vi "test29-MappingRelationshipByExternalRegistration_State.vi"(8 "error in (no error)":errorcluster, 11 "TestCase in":refnum<class "testcase-CSMBroadcast.lvclass">) -> (0 "error out":errorcluster, 3 "TestCase out":refnum<class "testcase-CSMBroadcast.lvclass">)   [LabVIEW 2017, in "testcase-CSMBroadcast.lvclass"]
uses:
  testcase-CSMBroadcast.lvclass
  5f1321ef-d679-4204-8b32-271554a776bf.vi
  3afc563d-56e9-48a4-901d-19be23a22e68.vi
  src/user.lib/_NEVSTOP/Communicable State Machine(CSM)/AdvanceAPI/CSM - Revert Arguments-Safe String.vi
  src/user.lib/_NEVSTOP/Communicable State Machine(CSM)/AdvanceAPI/CSM - Make String Arguments Safe.vi
  src/user.lib/_NEVSTOP/Communicable State Machine(CSM)/AdvanceAPI/CSM - Break Down Multiple States String.vi
  src/user.lib/_NEVSTOP/Communicable State Machine(CSM)/AdvanceAPI/CSM - Keywords.vi
  src/user.lib/_NEVSTOP/Communicable State Machine(CSM)/_Polymophic/CSM - Replace Marks in Messages.vi
  src/user.lib/_NEVSTOP/Communicable State Machine(CSM)/_Shared/Trim Single-line Text.vi
  src/user.lib/_NEVSTOP/Communicable State Machine(CSM)/Communicable State Machine.lvlib
  <vilib>/addons/_JKI Toolkits/VI Tester/TestCase.llb/TestCase.lvclass
  C:/Program Files (x86)/National Instruments/LabVIEW 2017/vi.lib/addons/_JKI Toolkits/VI Tester/TestCase.llb/TestCase.lvclass
panel:
  out "State History 2":string
  out "Loop Count":i32
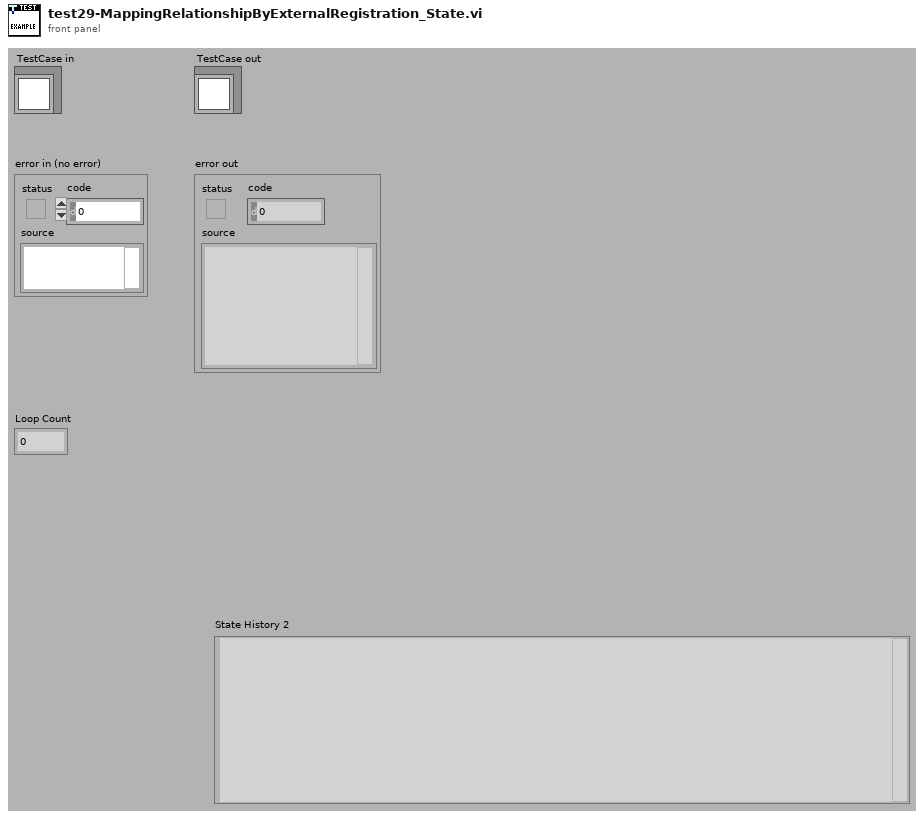
[diagram p1: front panel]
types:
  T1 = enum32{"Invalid", "Standard", "Closed", "Hidden", "Minimized", "Maximized"}
  T2 = enum32{"invalid app kind", "Development System", "Run Time System", "Student Edition", "Embedded LabVIEW", "Evaluation", "Custom"}
  T3 = cluster{"Status":string, "Source CSM":string, "Target CSM":string, "Target API":string}[]
  T4 = typedef "Communicable State Machine.lvlib/_CSM_Response Source Message.ctl" = cluster{"‘State":string, "’Arguments":string, "’Error":errorcluster}
  T5 = cluster{"Current VI Reference":refnum<vi>, "Close Panel on Exit?":bool}
  T6 = cluster{"Core":cluster{"Current VI Reference":refnum<vi>, "Close Panel on Exit?":bool}, "Your Boolean data":bool, "Your string data":string}
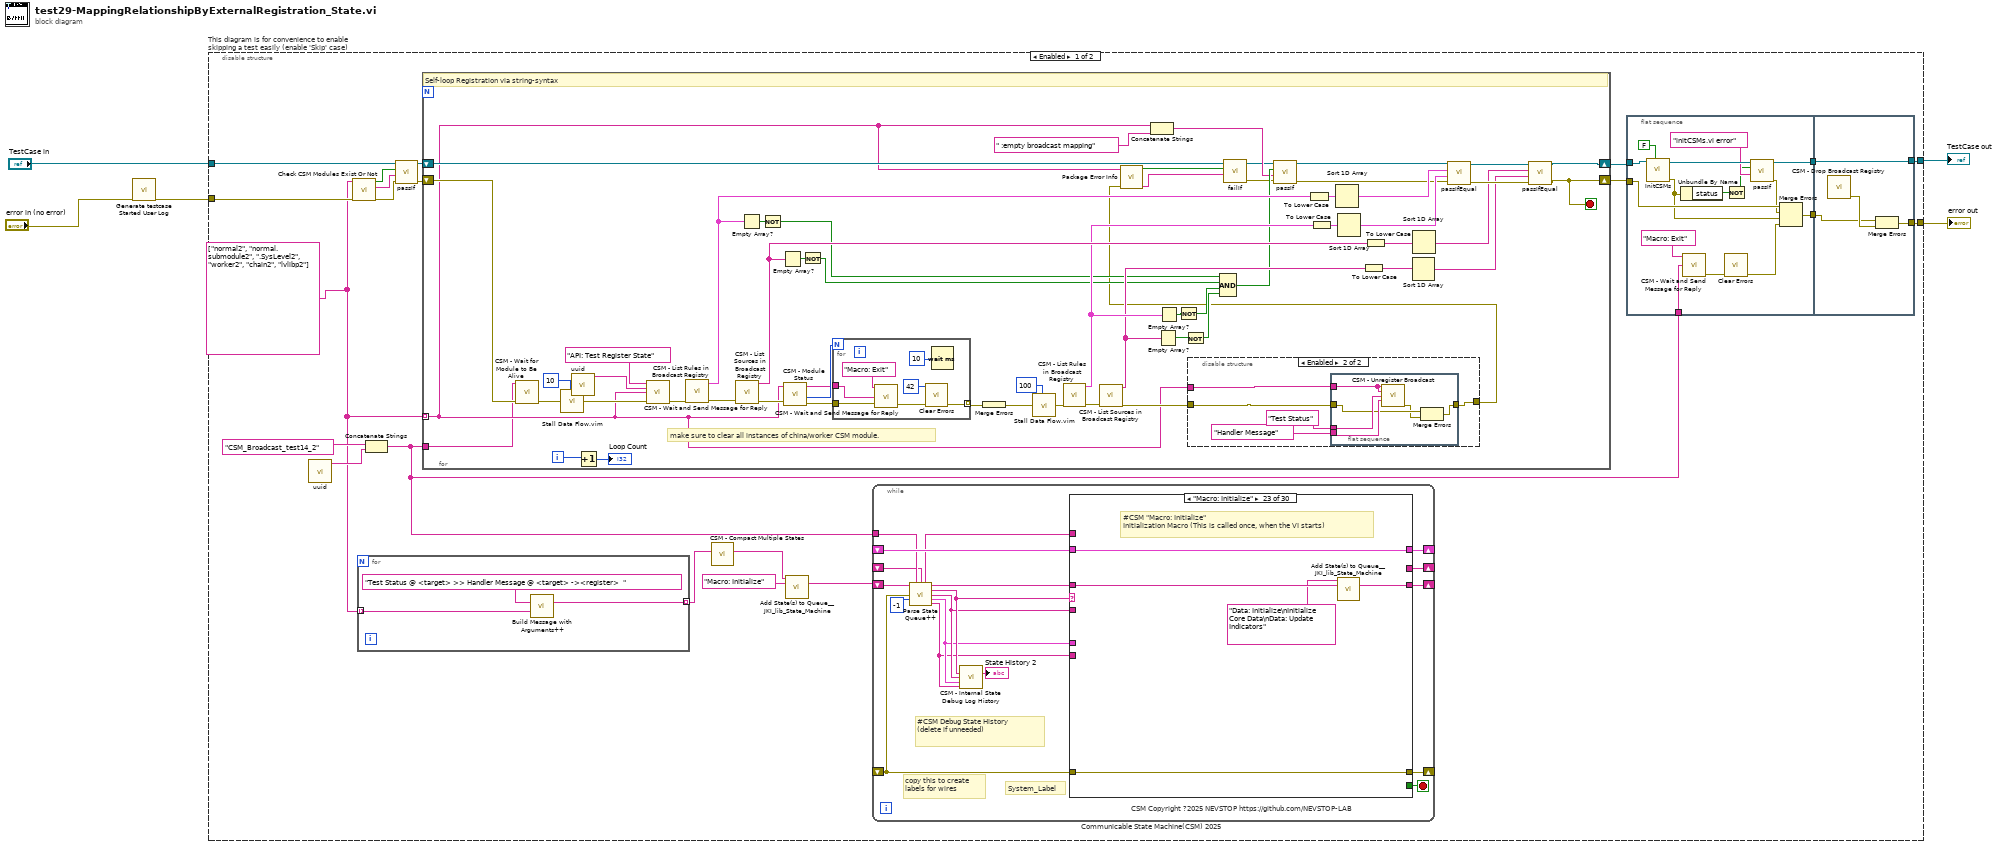
[diagram p0: block diagram]
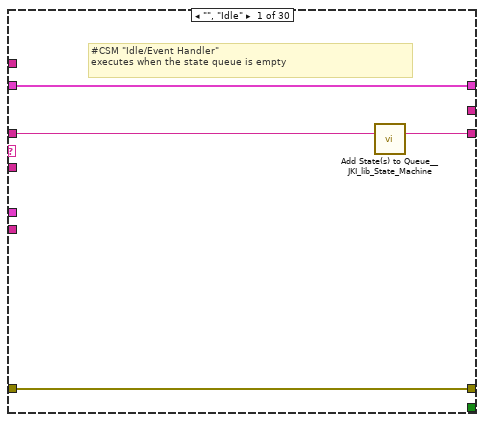
[diagram p2: hidden frame]
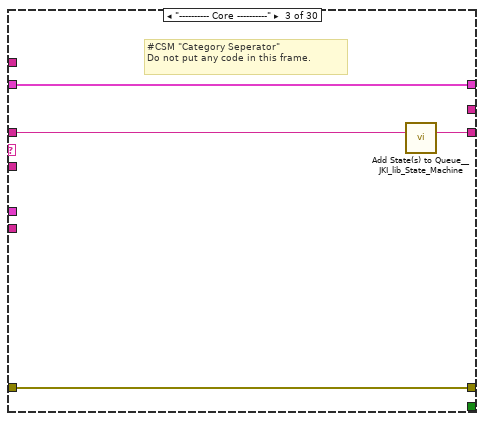
[diagram p4: hidden frame]
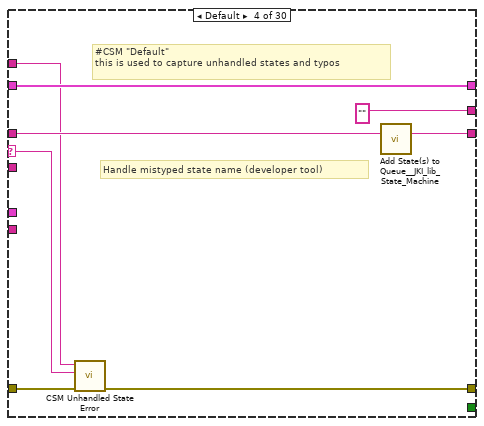
[diagram p5: hidden frame]
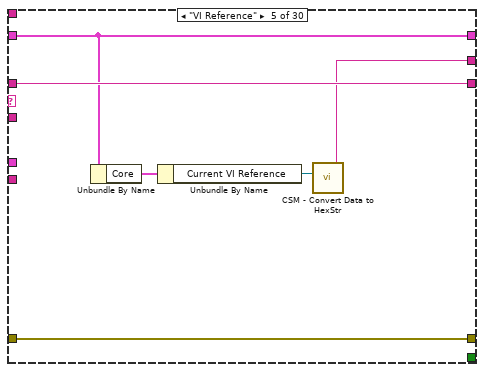
[diagram p6: hidden frame]
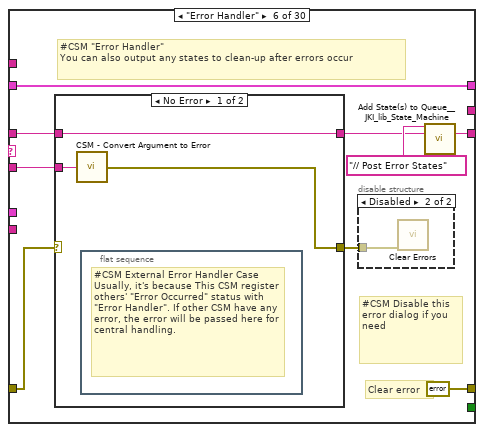
[diagram p7: hidden frame]
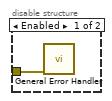
[diagram p8: hidden frame]
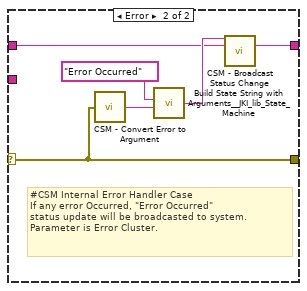
[diagram p9: hidden frame]
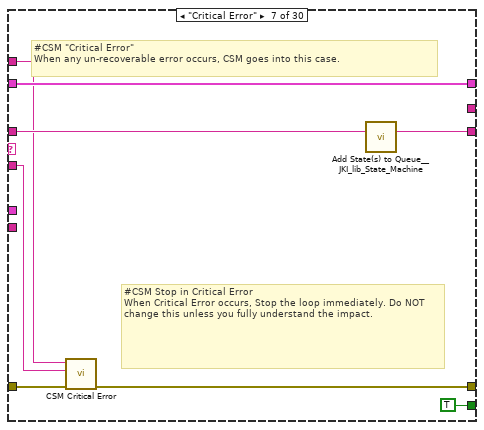
[diagram p10: hidden frame]
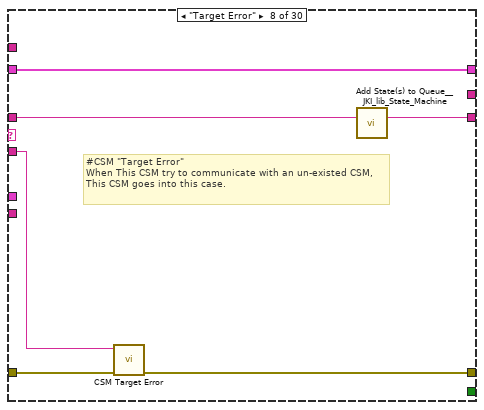
[diagram p11: hidden frame]
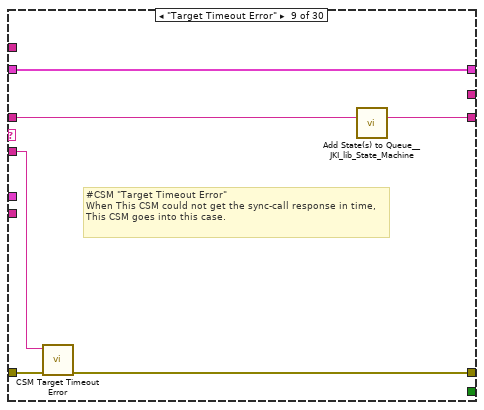
[diagram p12: hidden frame]
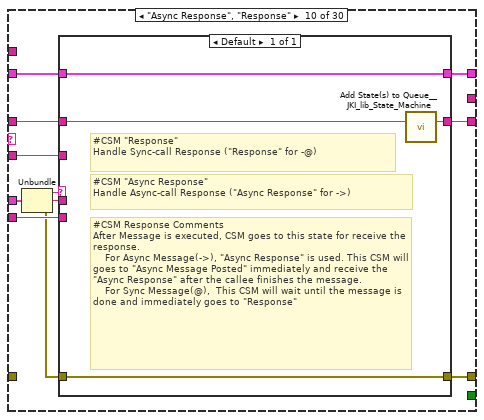
[diagram p13: hidden frame]
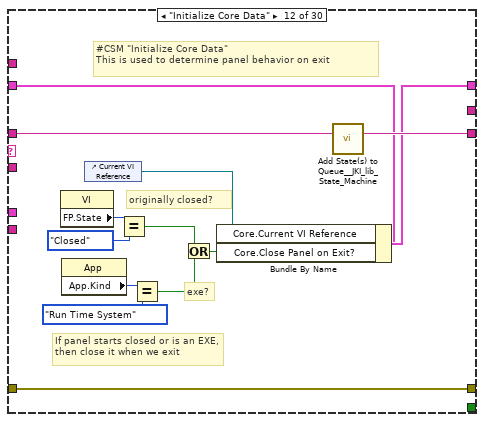
[diagram p15: hidden frame]
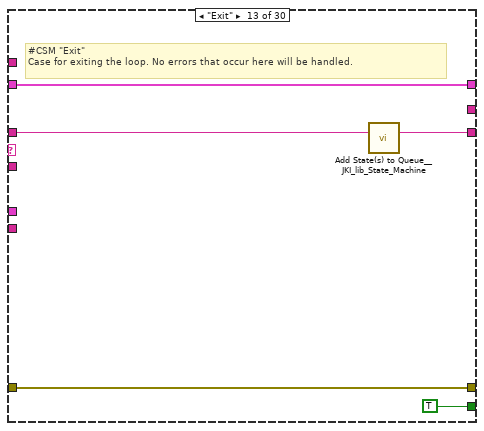
[diagram p16: hidden frame]
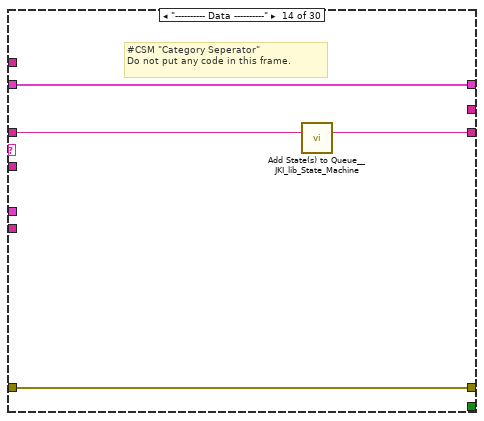
[diagram p17: hidden frame]
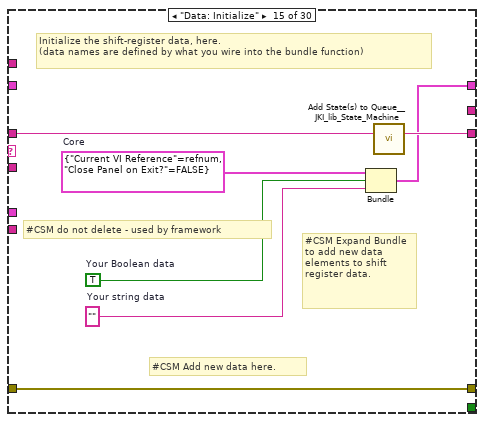
[diagram p18: hidden frame]
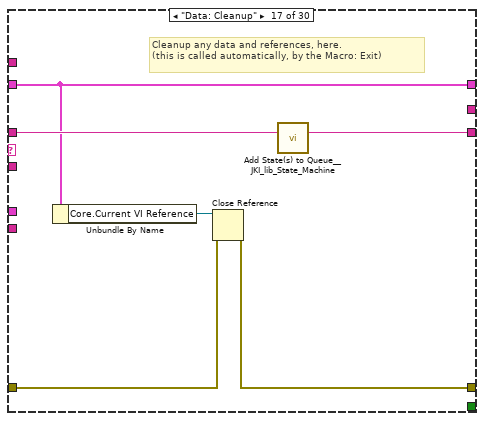
[diagram p20: hidden frame]
diagram:
  n1 = call "Generate testcase Started User Log.vi"("Error In"="error in (no error)") -> ("error out"=w1:errorcluster)  [unwired: 10 in]
  n2 = disable-structure "This diagram is for convenience to enable skipping a test easily (enable 'Skip' case)" shown="Enabled" {
    disable-tunnel: "TestCase in" -> [w21 w405]
    disable-tunnel: [w15 w403] -> w2
    disable-tunnel: [w14 w404] -> w4
    disable-tunnel: w1 -> [w23 w402]
    frame Enabled {
      w6 = string[] ["normal2", "normal.submodule2", ".SysLevel2", "worker2", "chain2", "lvlibp2"]
      n3 = call "uuid.vi"() -> ("UUID"=w8:string)  [unwired: 11 in]
      n4 = call "Check CSM Modules Exist Or Not.vi"("error in"=w23, "CSM names in"=w6) -> ("error out"=w24:errorcluster, "Debug string"=w25:string, "All Modules Exist?"=w26:bool)  [unwired: 7 in]
      n5 = for {
        tunnel: w6 -> [w28] mode=indexing
        tunnel: [w27] -> w11 mode=indexing
        n6 = call-poly "Build Message with Arguments++.vi"("States With Replace Token"="Test Status @ <target> >> Handler Message @ <target> -><register>  " ("State"), "<target>"=w28) -> ("States"=w27:string)  [unwired: 13 in]
      }
      n7 = Concatenate Strings("CSM_Broadcast_test14_2" ("Name (\"\" to Use UUID)"), w8) -> (w7:string)
      n8 = call-dynamic "passIf.vi"("error in (no error)"=w24, "message (\"\")"=w25, "pass"=w26, "TestCase in"=w21) -> ("error out"=w22:errorcluster, "TestCase out"=w20:refnum<class "testcase-CSMBroadcast.lvclass">)  [unwired: 6 in]
      n9 = for {
        tunnel: w6 -> [w330] mode=indexing
        shift-right: [w325] -> w17
        shift-left: w20 -> [w335]
        shift-right: [w324] -> w16
        shift-left: w22 -> [w341]
        tunnel: w7 -> [w327]
        i -> [w364]
        stop <- w324 stop-if-true
        # "make sure to clear all instances of china/worker CSM module."
        # "Self-loop Registration via string-syntax"
        n10 = call "CSM - Wait for Module to Be Alive.vi"("CSM Name"=w327, "error in (no error)"=w341) -> ("error out"=w349:errorcluster)  [unwired: 11 in, 2 out]
        n11 = call "Stall Data Flow.vim"("value in"=w349, "milliseconds to wait"=u32 10) -> ("value out"=w348:errorcluster)  [unwired: 1 out]
        n12 = call "uuid.vi"() -> ("UUID"=w379:string)  [unwired: 11 in]
        n13 = Increment(x=w364) -> (x+1=→"Loop Count":i32)
        n14 = call "CSM - Wait and Send Message for Reply.vi"("State"="API: Test Register State", "Arguments (\"\")"=w379, "Target Module"=w330, "Error In (No Error)"=w348) -> ("error out"=w378:errorcluster)  [unwired: 8 in, 3 out]
        n15 = call "CSM - List Rules in Broadcast Registry.vi"("error in (no error)"=w378) -> ("error out"=w376:errorcluster, "Rule Entries"=w362:T3)  [unwired: 8 in, 1 out]
        n16 = call "CSM - List Sources in Broadcast Registry.vi"("error in (no error)"=w376) -> ("error out"=w343:errorcluster, "Broadcast Names"=w359:string[])  [unwired: 9 in]
        n17 = Empty Array?(array=w362) -> (empty?=w361:bool)
        n18 = Not(x=w361) -> (.not. x?=w354:bool)
        n19 = Empty Array?(array=w359) -> (empty?=w360:bool)
        n20 = call "CSM - Module Status.vi"("Error In"=w343, "CSM Name"=w330) -> ("error out"=w344:errorcluster, "#Nodes"=w346:i32, "CSM Name (Dup)"=w345:string)  [unwired: 5 in, 2 out]
        n21 = Not(x=w360) -> (.not. x?=w353:bool)
        n22 = for {
          N: w346 -> [_]
          tunnel: w345 -> [w386]
          tunnel: w344 -> [w384]
          tunnel: [w383] -> w377 mode=indexing
          n23 = call "CSM - Wait and Send Message for Reply.vi"("State"="Macro: Exit", "Target Module"=w386, "Error In (No Error)"=w384) -> ("error out"=w385:errorcluster)  [unwired: 9 in, 3 out]
          n24 = call <vilib>:"Clear Errors.vi"("error in (no error)"=w385, "specific error code to clear (0: all)"=42) -> ("error out"=w383:errorcluster)  [unwired: 4 in, 1 out]
          n25 = Wait (ms)(milliseconds to wait=u32 10) -> ()  [unwired: 1 out]
        }
        n26 = Merge Errors(w377) -> (w332:errorcluster)
        n27 = call "Stall Data Flow.vim"("value in"=w332, "milliseconds to wait"=u32 100) -> ("value out"=w331:errorcluster)  [unwired: 1 out]
        n28 = call "CSM - List Rules in Broadcast Registry.vi"("error in (no error)"=w331) -> ("error out"=w375:errorcluster, "Rule Entries"=w357:T3)  [unwired: 8 in, 1 out]
        n29 = call "CSM - List Sources in Broadcast Registry.vi"("error in (no error)"=w375) -> ("error out"=w352:errorcluster, "Broadcast Names"=w355:string[])  [unwired: 9 in]
        n30 = Concatenate Strings(w330, " :empty broadcast mapping" ("string")) -> (w337:string)
        n31 = Empty Array?(array=w355) -> (empty?=w356:bool)
        n32 = Empty Array?(array=w357) -> (empty?=w358:bool)
        n33 = Not(x=w358) -> (.not. x?=w351:bool)
        n34 = Not(x=w356) -> (.not. x?=w350:bool)
        n35 = disable-structure shown="Enabled" {
          disable-tunnel: w352 -> [w390 w394]
          disable-tunnel: w330 -> [w389 w395]
          disable-tunnel: [w388 w393] -> w326
          frame Disabled {
            n36 = call "CSM - Remove Module in Broadcast Registry.vi"("CSM Name"=w389, "Error In"=w390) -> ("error out"=w388:errorcluster)  [unwired: 12 in, 1 out]
          }
          frame Enabled {
            n37 = flat-sequence {
              tunnel: "Test Status" ("Status") -> [w401]
              tunnel: "Handler Message" ("Response Message (If \"\", Same as Source Message)") -> [w400]
              tunnel: w395 -> [w399]
              tunnel: w394 -> [w398]
              tunnel: [w396] -> w393
              frame #0 {
                n38 = call "CSM - Unregister Broadcast.vi"("CSM Name(Empty for Broadcast Event)"=w399, "Source CSM Name (* as Default)"=w399, "Trigger"=w401, "API (\"*\" as Default)"=w400) -> ("error out"=w397:errorcluster)  [unwired: 10 in, 1 out]
                n39 = Merge Errors(w398, w397) -> (w396:errorcluster)
              }
            }
          }
        }
        n40 = call "Package Error Info.vi"("error in"=w326, "String in"=w330) -> ("packed error info out"=w328:string, "error status"=w329:bool)  [unwired: 8 in]
        n41 = Compound Arithmetic op=AND(w354, w353, w351, w350) -> (w339:bool)
        n42 = call-dynamic "failIf.vi"("message (\"\")"=w328, "fail"=w329, "TestCase in"=w335) -> ("error out"=w334:errorcluster, "TestCase out"=w336:refnum<class "testcase-CSMBroadcast.lvclass">)  [unwired: 7 in]
        n43 = call-dynamic "passIf.vi"("error in (no error)"=w334, "message (\"\")"=w337, "pass"=w339, "TestCase in"=w336) -> ("error out"=w340:errorcluster, "TestCase out"=w342:refnum<class "testcase-CSMBroadcast.lvclass">)  [unwired: 6 in]
        n44 = To Lower Case(string=w362) -> (all lower case string=w374:T3)
        n45 = To Lower Case(string=w357) -> (all lower case string=w373:T3)
        n46 = Sort 1D Array(array=w374) -> (sorted array=w372:T3)
        n47 = Sort 1D Array(array=w373) -> (sorted array=w371:T3)
        n48 = To Lower Case(string=w355) -> (all lower case string=w367:string[])
        n49 = To Lower Case(string=w359) -> (all lower case string=w368:string[])
        n50 = Sort 1D Array(array=w367) -> (sorted array=w365:string[])
        n51 = Sort 1D Array(array=w368) -> (sorted array=w366:string[])
        n52 = call-dynamic "passIfEqual.vi"("error in (no error)"=w340, "y"=w371, "x"=w372, "TestCase in"=w342) -> ("error out"=w369:errorcluster, "TestCase out"=w370:refnum<class "testcase-CSMBroadcast.lvclass">)  [unwired: 6 in]
        n53 = call-dynamic "passIfEqual.vi"("error in (no error)"=w369, "y"=w365, "x"=w366, "TestCase in"=w370) -> ("error out"=w324:errorcluster, "TestCase out"=w325:refnum<class "testcase-CSMBroadcast.lvclass">)  [unwired: 6 in]
      }
      n54 = call "CSM - Compact Multiple States.vi"("Multiple States"=w11) -> ("States"=w10:string)  [unwired: 9 in]
      n55 = call <vilib>:"Add State(s) to Queue__JKI_lib_State_Machine.vi"("State(s) in Front (\"\")"=w10, "State(s) in (\"\")"="Macro: Initialize" ("Init State(\"Macro: Initialize\")")) -> ("States Out"=w12:string)  [unwired: 13 in]
      n56 = while "Communicable State Machine(CSM) 2025" {
        shift-right: [w42] -> _
        shift-left: _ -> [w41]
        shift-right: [w45] -> _
        shift-left: _ -> [w40]
        shift-right: [w44] -> _
        shift-left: w12 -> [w46]
        tunnel: w7 -> [w38]
        shift-right: [w39] -> _
        shift-left: _ -> [w32]
        stop <- w43 stop-if-true
        # "#CSM Debug State History\n(delete if unneeded)"
        # "copy this to create labels for wires"
        # "System_Label"
        # "CSM Copyright ?2025 NEVSTOP https://github.com/NEVSTOP-LAB"
        n57 = call "Parse State Queue++.vi"("State Queue"=w46, "Name (\"\" to Use UUID)"=w38, "Response Arguments"=w32, "Previous Error"=w40, "Dequeue (1 ms)"=-1 ("Timeout")) -> ("Name Used"=w33:string, "Remaining States"=w47:string, "Current State"=w37:string, "Arguments"=w36:string, "Additional Information"=w35:T4, "Source CSM"=w34:string)  [unwired: 5 in]
        n58 = call "CSM - Internal State Debug Log History.vi"("State"=w37, "Arguments (\"\")"=w36, ">> Response Source Message >>"=w35, "Source (\"\")"=w34) -> ("Debug Log"=→"State History 2":string)  [unwired: 11 in]
        n59 = case shown="\"Macro: Initialize\"" w37 {
          selector: w37 -> [_ _ _ w61 _ _ _ _ _ _ _ _ _ _ _ _ _ _ _ _ _ _ _ _ _ _ _ _ _ _]
          tunnel: w47 -> [w48 w53 w58 w65 w71 w77 w98 w104 w110 w118 w129 w143 w148 w152 w159 w161 w168 w172 w176 w182 w197 w266 w271 w278 w280 w284 w289 w296 w300 w304]
          tunnel: w36 -> [_ _ _ _ _ w76 w94 w103 w108 w117 _ _ _ _ _ _ _ _ _ w177 w191 _ _ _ _ _ w287 _ _ _]
          tunnel: w41 -> [w49 w52 w55 w63 w70 w80 w99 w105 w111 w120 w128 w136 w146 w149 _ w160 w163 w169 w174 w180 w193 w263 w268 w275 w279 w283 w288 w293 w297 w301]
          tunnel: [w50 w54 w56 w59 w72 errorcluster {"status"=FALSE, "code"=0, "source"=""} ("error out") w95 w101 w107 w123 w130 w140 w145 w150 w156 w162 w164 w170 w173 w178 w194 w264 w269 w276 w281 w285 w290 w294 w298 w302] -> w45
          tunnel: w40 -> [w50 w54 w56 w66 w72 w78 w100 w102 w109 _ w130 w140 w145 w150 w156 w162 w165 w170 w173 w179 w195 w264 w269 w276 w281 w285 w290 w294 w298 w302]
          tunnel: [w51 w53 w57 w64 w71 w73 w97 w106 w112 w119 w129 w142 w147 w151 w158 w161 w167 w171 w175 w181 w196 w265 w270 w277 w280 w284 w289 w295 w299 w303] -> w44
          tunnel: [_ _ _ _ _ _ TRUE _ _ _ _ _ TRUE _ _ _ _ _ _ _ _ _ _ _ _ _ _ _ _ _] -> w43
          tunnel: [w49 w52 w55 w63 w70 w80 w99 w105 w111 w121 w128 w141 w146 w149 w157 w160 w163 w169 w174 w180 w193 w263 w268 w275 w279 w283 w288 w293 w297 w301] -> w42
          tunnel: w34 -> [_ _ _ _ _ _ _ _ _ w115 _ _ _ _ _ _ _ _ _ _ _ _ _ _ _ _ _ _ _ _]
          tunnel: w35 -> [_ _ _ _ _ _ _ _ _ w122 _ _ _ _ _ _ _ _ _ _ _ _ _ _ _ _ _ _ _ _]
          tunnel: [_ _ _ "" w67 _ _ _ _ _ _ _ _ _ _ _ _ _ _ _ _ _ _ _ _ "API1 Response" w286 _ _ _] -> w39
          tunnel: w33 -> [_ _ _ w60 _ _ w93 _ _ _ _ _ _ _ _ _ _ _ _ _ _ _ _ _ _ _ _ _ _ _]
          frame "", "Idle" {
            # "#CSM \"Idle/Event Handler\"\nexecutes when the state queue is empty"
            n60 = call <vilib>:"Add State(s) to Queue__JKI_lib_State_Machine.vi"("State(s) in (\"\")"=w48) -> ("States Out"=w51:string)  [unwired: 14 in]
          }
          frame "CSM Documentation" {
            # "#CSM README FIRST\n\nCommunicable State Machine(CSM) is a LabVIEW application framework that builds upon JKI State Machine(JKISM). It follows the pattern of JKISM and extends the keywords to describe message communication between modules, including concepts such as Sync-Message, Async-Message, Subscription/Unsubscription of status - essential elements for creating reusable code modules. For more information, please visit the CSM wiki: https://nevstop-lab.github.io/CSM-Wiki/\n\nFor instructions on JKI State Machine, visit: http://jki.net/state-machine/\nFor information about CSM, visit: https://github.com/NEVSTOP-LAB"
            # "#CSM \"Documentation\"\nCase for holding CSM Documenation"
          }
          frame "---------- Core ----------" {
            # "#CSM \"Category Seperator\"\nDo not put any code in this frame."
            n61 = call <vilib>:"Add State(s) to Queue__JKI_lib_State_Machine.vi"("State(s) in (\"\")"=w58) -> ("States Out"=w57:string)  [unwired: 14 in]
          }
          frame Default {
            # "#CSM \"Default\"\nthis is used to capture unhandled states and typos"
            # "Handle mistyped state name (developer tool)"
            n62 = call "CSM Unhandled State Error.vi"("error in (no error)"=w66, "Undefined State"=w61, "CSM Name"=w60) -> ("error out"=w59:errorcluster)  [unwired: 8 in]
            n63 = call <vilib>:"Add State(s) to Queue__JKI_lib_State_Machine.vi"("State(s) in (\"\")"=w65) -> ("States Out"=w64:string)  [unwired: 14 in]
          }
          frame "VI Reference" {
            n64 = Unbundle By Name(w70) -> ("Core"=w69:T5)
            n65 = Unbundle By Name(w69) -> ("Current VI Reference"=w68:refnum<vi>)
            n66 = call "CSM - Convert Data to HexStr.vi"("Variant"=w68) -> ("HEX String (0-9,A-F)"=w67:string)  [unwired: 8 in]
          }
          frame "Error Handler" {
            # "#CSM Disable this error dialog if you need"
            # "#CSM \"Error Handler\"\nYou can also output any states to clean-up after errors occur"
            # "Clear error"
            n67 = case shown="No Error" w78 {
              selector: w78 -> [_ w87]
              tunnel: [w86 w89] -> w74
              tunnel: w77 -> [w86 w88]
              tunnel: w76 -> [w85 _]
              tunnel: [w84 w87] -> w79
              frame No Error {
                n68 = call "CSM - Convert Argument to Error.vi"("Argument"=w85) -> ("Error"=w84:errorcluster)  [unwired: 4 in]
                n69 = flat-sequence {
                  frame #0 {
                    # "#CSM External Error Handler Case\nUsually, it's because This CSM register others' \"Error Occurred\" status with \"Error Handler\". If other CSM have any error, the error will be passed here for central handling."
                  }
                }
              }
              frame Error {
                # "#CSM Internal Error Handler Case \nIf any error Occurred, \"Error Occurred\" \nstatus update will be broadcasted to system.\nParameter is Error Cluster."
                n70 = call "CSM - Convert Error to Argument.vi"("Error"=w87) -> ("Argument"=w91:string)  [unwired: 4 in]
                n71 = call <vilib>:"Build State String with Arguments__JKI_lib_State_Machine.vi"("Arguments (\"\")"=w91, "State"="Error Occurred" ("Status with Arguments")) -> ("State with Arguments"=w90:string)  [unwired: 4 in]
                n72 = call "CSM - Broadcast Status Change.vi"("Status With Arguments"=w90, "State Queue"=w88) -> ("Remaining States"=w89:string)  [unwired: 13 in]
              }
            }
            n73 = disable-structure shown="Disabled" {
              disable-tunnel: w79 -> [w82 w83]
              frame Enabled {
                n74 = call <vilib>:"General Error Handler.vi"("error in (no error)"=w82) -> ()  [unwired: 10 in, 5 out]
              }
              frame Disabled {
                n75 = call <vilib>:"Clear Errors.vi"("error in (no error)"=w83) -> ()  [unwired: 5 in, 2 out]
              }
            }
            n76 = call <vilib>:"Add State(s) to Queue__JKI_lib_State_Machine.vi"("State(s) in Front (\"\")"="// Post Error States", "State(s) in (\"\")"=w74) -> ("States Out"=w73:string)  [unwired: 13 in]
          }
          frame "Critical Error" {
            # "#CSM Stop in Critical Error\nWhen Critical Error occurs, Stop the loop immediately. Do NOT change this unless you fully understand the impact."
            # "#CSM \"Critical Error\"\nWhen any un-recoverable error occurs, CSM goes into this case."
            n77 = call "CSM Critical Error.vi"("error in (no error)"=w100, "Arugments (As Reason)"=w94, "CSM Name"=w93) -> ("error out"=w95:errorcluster)  [unwired: 8 in]
            n78 = call <vilib>:"Add State(s) to Queue__JKI_lib_State_Machine.vi"("State(s) in (\"\")"=w98) -> ("States Out"=w97:string)  [unwired: 14 in]
          }
          frame "Target Error" {
            # "#CSM \"Target Error\"\nWhen This CSM try to communicate with an un-existed CSM, This CSM goes into this case."
            n79 = call "CSM Target Error.vi"("error in (no error)"=w102, "Arguments (As CSM Name)"=w103) -> ("error out"=w101:errorcluster)  [unwired: 9 in]
            n80 = call <vilib>:"Add State(s) to Queue__JKI_lib_State_Machine.vi"("State(s) in (\"\")"=w104) -> ("States Out"=w106:string)  [unwired: 14 in]
          }
          frame "Target Timeout Error" {
            # "#CSM \"Target Timeout Error\"\nWhen This CSM could not get the sync-call response in time, This CSM goes into this case."
            n81 = call "CSM Target Timeout Error.vi"("error in (no error)"=w109, "Arguments (As CSM Name)"=w108) -> ("error out"=w107:errorcluster)  [unwired: 9 in]
            n82 = call <vilib>:"Add State(s) to Queue__JKI_lib_State_Machine.vi"("State(s) in (\"\")"=w110) -> ("States Out"=w112:string)  [unwired: 14 in]
          }
          frame "Async Response", "Response" {
            n83 = Unbundle(w122) -> ("‘State"=w116:string, "’Arguments"=w114:string, "’Error"=w113:errorcluster)
            n84 = case shown="Default" w116 {
              tunnel: [w127] -> w123
              tunnel: w113 -> [w127]
              tunnel: [w126] -> w121
              tunnel: w120 -> [w126]
              tunnel: [w124] -> w119
              tunnel: w118 -> [w125]
              tunnel: w117 -> [_]
              tunnel: w115 -> [_]
              tunnel: w114 -> [_]
              frame Default {
                # "#CSM Response Comments\nAfter Message is executed, CSM goes to this state for receive the response.\n    For Async Message(->), \"Async Response\" is used. This CSM will goes to \"Async Message Posted\" immediately and receive the \"Async Response\" after the callee finishes the message.\n    For Sync Message(@),  This CSM will wait until the message is done and immediately goes to \"Response\""
                # "#CSM \"Async Response\"\nHandle Async-call Response (\"Async Response\" for ->)"
                # "#CSM \"Response\"\nHandle Sync-call Response (\"Response\" for -@)"
                n85 = call <vilib>:"Add State(s) to Queue__JKI_lib_State_Machine.vi"("State(s) in (\"\")"=w125) -> ("States Out"=w124:string)  [unwired: 14 in]
              }
            }
          }
          frame "Async Message Posted" {
            # "#CSM \"Async Message Posted\"\nAfter Async Message is posted (-> or ->| ), CSM goes to this state for post-action.\nYou can use Argument - State to tell which Async Message is called."
          }
          frame "Initialize Core Data" {
            # "#CSM \"Initialize Core Data\"\nThis is used to determine panel behavior on exit"
            # "originally closed?"
            # "exe?"
            # "If panel starts closed or is an EXE, then close it when we exit"
            n86 = property class="VI"() -> ("FP.State"=w133:T1)  [unwired: 2 in, 2 out]
            n87 = property class="App"() -> ("App.Kind"=w139:T2)  [unwired: 2 in, 2 out]
            n88 = control-ref of="Current VI Reference"() -> (w134:refnum<vi>)
            n89 = Equal?(x=w133, y=T1."Closed" ("Front Panel Window:State")) -> (x = y?=w131:bool)
            n90 = Equal?(x=w139, y=T2."Run Time System" ("Application:Kind")) -> (x = y?=w137:bool)
            n91 = Or(x=w131, y=w137) -> (x .or. y?=w135:bool)
            n92 = Bundle By Name(cluster=w136, "Core.Current VI Reference"=w134, "Core.Close Panel on Exit?"=w135) -> (w141:T6)
            n93 = call <vilib>:"Add State(s) to Queue__JKI_lib_State_Machine.vi"("State(s) in (\"\")"=w143) -> ("States Out"=w142:string)  [unwired: 14 in]
          }
          frame "Exit" {
            # "#CSM \"Exit\"\nCase for exiting the loop. No errors that occur here will be handled."
            n94 = call <vilib>:"Add State(s) to Queue__JKI_lib_State_Machine.vi"("State(s) in (\"\")"=w148) -> ("States Out"=w147:string)  [unwired: 14 in]
          }
          frame "---------- Data ----------" {
            # "#CSM \"Category Seperator\"\nDo not put any code in this frame."
            n95 = call <vilib>:"Add State(s) to Queue__JKI_lib_State_Machine.vi"("State(s) in (\"\")"=w152) -> ("States Out"=w151:string)  [unwired: 14 in]
          }
          frame "Data: Initialize" {
            w153 = T5 {"Current VI Reference"=refnum, "Close Panel on Exit?"=FALSE}  # Core
            w155 = TRUE  # Your Boolean data
            w154 = ""  # Your string data
            # "#CSM do not delete - used by framework"
            # "#CSM Expand Bundle to add new data elements to shift register data."
            # "#CSM Add new data here."
            # "Initialize the shift-register data, here.\n(data names are defined by what you wire into the bundle function)"
            n96 = Bundle("Core"=w153, "Your Boolean data"=w155, "Your string data"=w154) -> (w157:T6)  [unwired: 1 in]
            n97 = call <vilib>:"Add State(s) to Queue__JKI_lib_State_Machine.vi"("State(s) in (\"\")"=w159) -> ("States Out"=w158:string)  [unwired: 14 in]
          }
          frame "Data: Update Indicators" {
          }
          frame "Data: Cleanup" {
            # "Cleanup any data and references, here.\n(this is called automatically, by the Macro: Exit)"
            n98 = Unbundle By Name(w163) -> ("Core.Current VI Reference"=w166:refnum<vi>)
            n99 = Close Reference(reference=w166, error in (no error)=w165) -> (error out=w164:errorcluster)
            n100 = call <vilib>:"Add State(s) to Queue__JKI_lib_State_Machine.vi"("State(s) in (\"\")"=w168) -> ("States Out"=w167:string)  [unwired: 14 in]
          }
          frame "---------- UI ----------" {
            # "#CSM \"Category Seperator\"\nDo not put any code in this frame."
            n101 = call <vilib>:"Add State(s) to Queue__JKI_lib_State_Machine.vi"("State(s) in (\"\")"=w172) -> ("States Out"=w171:string)  [unwired: 14 in]
          }
          frame "UI: Initialize" {
            # "#CSM \"UI: Initialize\"\nInitialize the User Interface, here.\n(this is called automatically, by the Macro: Init)"
            n102 = call <vilib>:"Add State(s) to Queue__JKI_lib_State_Machine.vi"("State(s) in (\"\")"=w176) -> ("States Out"=w175:string)  [unwired: 14 in]
          }
          frame "UI: Cursor Set" {
            # "#CSM \"UI: Cursor Set\"\nSet and Unset Cursor Busy.\n(Usage: \"UI: Cursor Set >> Busy|Idle\")"
            # "Argument"
            n103 = disable-structure shown="TARGET_TYPE!=Windows" {
              disable-tunnel: w179 -> [w185 w190]
              disable-tunnel: [w184 w190] -> w178
              disable-tunnel: w177 -> [w183 _]
              frame condition #0 (active) {
                n104 = case shown="\"Idle\", Default" w183 {
                  tunnel: w185 -> [w187 w189]
                  tunnel: [w186 w188] -> w184
                  frame "Idle", Default {
                    n105 = call <vilib>:"Unset Busy.vi"("error in (no error)"=w187) -> ("error out"=w186:errorcluster)  [unwired: 10 in]
                  }
                  frame "Busy" {
                    n106 = call <vilib>:"Set Busy.vi"("error in (no error)"=w189) -> ("error out"=w188:errorcluster)  [unwired: 9 in, 1 out]
                  }
                }
              }
              frame condition #1 {
              }
            }
            n107 = call <vilib>:"Add State(s) to Queue__JKI_lib_State_Machine.vi"("State(s) in (\"\")"=w182) -> ("States Out"=w181:string)  [unwired: 14 in]
          }
          frame "UI: Front Panel State" {
            # "#CSM \"UI: Front Panel State\"\nSet Front Panel Open or Closed\n(Usage: \"UI: Front Panel State >> Open|Close\")"
            # "Argument"
            n108 = Unbundle By Name(w193) -> ("Core.Current VI Reference"=w192:refnum<vi>)
            n109 = call <vilib>:"Add State(s) to Queue__JKI_lib_State_Machine.vi"("State(s) in (\"\")"=w197) -> ("States Out"=w196:string)  [unwired: 14 in]
            n110 = case shown="\"Close\", \"Closed\"" w191 {
              tunnel: w195 -> [w203 w218 w229 w242 w255]
              tunnel: [w205 w219 w231 w244 w257] -> w194
              tunnel: w192 -> [w204 w216 w230 w243 w256]
              frame "Open", "Standard", Default {
                w198 = T1."Standard" ("State")
                n111 = property class="VI"(reference=w204, error in=w203) -> (reference out=w201:refnum<vi>, error out=w202:errorcluster, "FP.State"=w200:T1)
                n112 = Not Equal?(x=w200, y=w198) -> (x != y?=w199:bool)
                n113 = case shown="True" w199 {
                  tunnel: [w209 w211] -> w205
                  tunnel: w202 -> [w208 w211]
                  tunnel: w201 -> [w207 _]
                  tunnel: w198 -> [w206 _]
                  frame True {
                    n114 = invoke class="VI" method="FP.Open"(reference=w207, error in=w208, "Activate"=TRUE, "State"=w206) -> (error out=w209:errorcluster)  [unwired: 1 in, 4 out]
                  }
                  frame False {
                  }
                }
              }
              frame "Close", "Closed" {
                n115 = property class="VI"(reference=w216, error in=w218) -> (reference out=w215:refnum<vi>, error out=w217:errorcluster, "FP.State"=w213:T1)
                n116 = Not Equal?(x=w213, y=T1."Closed" ("Front Panel Window:State")) -> (x != y?=w212:bool)
                n117 = case shown="False" w212 {
                  tunnel: [w220 w223] -> w219
                  tunnel: w217 -> [w220 w222]
                  tunnel: w215 -> [_ w221]
                  frame False {
                  }
                  frame True {
                    n118 = invoke class="VI" method="FP.Close"(reference=w221, error in=w222) -> (error out=w223:errorcluster)  [unwired: 1 in, 2 out]
                  }
                }
              }
              frame "Hidden", "Hide" {
                w224 = T1."Hidden" ("State")
                n119 = property class="VI"(reference=w230, error in=w229) -> (reference out=w227:refnum<vi>, error out=w228:errorcluster, "FP.State"=w226:T1)
                n120 = Not Equal?(x=w226, y=w224) -> (x != y?=w225:bool)
                n121 = case shown="True" w225 {
                  tunnel: [w235 w236] -> w231
                  tunnel: w228 -> [w234 w236]
                  tunnel: w227 -> [w233 _]
                  tunnel: w224 -> [w232 _]
                  frame True {
                    n122 = invoke class="VI" method="FP.Open"(reference=w233, error in=w234, "State"=w232) -> (error out=w235:errorcluster)  [unwired: 2 in, 4 out]
                  }
                  frame False {
                  }
                }
              }
              frame "Minimize", "Minimized" {
                w237 = T1."Minimized" ("State")
                n123 = property class="VI"(reference=w243, error in=w242) -> (reference out=w240:refnum<vi>, error out=w241:errorcluster, "FP.State"=w239:T1)
                n124 = Not Equal?(x=w239, y=w237) -> (x != y?=w238:bool)
                n125 = case shown="True" w238 {
                  tunnel: [w248 w249] -> w244
                  tunnel: w241 -> [w247 w249]
                  tunnel: w240 -> [w246 _]
                  tunnel: w237 -> [w245 _]
                  frame True {
                    n126 = invoke class="VI" method="FP.Open"(reference=w246, error in=w247, "State"=w245) -> (error out=w248:errorcluster)  [unwired: 2 in, 4 out]
                  }
                  frame False {
                  }
                }
              }
              frame "Maximize", "Maximized" {
                w250 = T1."Maximized" ("State")
                n127 = property class="VI"(reference=w256, error in=w255) -> (reference out=w253:refnum<vi>, error out=w254:errorcluster, "FP.State"=w252:T1)
                n128 = Not Equal?(x=w252, y=w250) -> (x != y?=w251:bool)
                n129 = case shown="True" w251 {
                  tunnel: [w261 w262] -> w257
                  tunnel: w254 -> [w260 w262]
                  tunnel: w253 -> [w259 _]
                  tunnel: w250 -> [w258 _]
                  frame True {
                    n130 = invoke class="VI" method="FP.Open"(reference=w259, error in=w260, "State"=w258) -> (error out=w261:errorcluster)  [unwired: 2 in, 4 out]
                  }
                  frame False {
                  }
                }
              }
            }
          }
          frame "---------- Macro ----------" {
            # "#CSM \"Category Seperator\"\nDo not put any code in this frame."
            n131 = call <vilib>:"Add State(s) to Queue__JKI_lib_State_Machine.vi"("State(s) in (\"\")"=w266) -> ("States Out"=w265:string)  [unwired: 14 in]
          }
          frame "Macro: Initialize" {
            # "#CSM \"Macro: Initialize\"\nInitialization Macro (This is called once, when the VI starts)"
            n132 = call <vilib>:"Add State(s) to Queue__JKI_lib_State_Machine.vi"("State(s) in Front (\"\")"="Data: Initialize\nInitialize Core Data\nData: Update Indicators", "State(s) in (\"\")"=w271) -> ("States Out"=w270:string)  [unwired: 13 in]
          }
          frame "Macro: Exit" {
            # "#CSM \"Macro: Exit\"\nExit Macro (This is called once, when the VI exits)"
            n133 = call <vilib>:"Add State(s) to Queue__JKI_lib_State_Machine.vi"("State(s) in Front (\"\")"="//Exit Sub-Modules ", "State(s) at Back (\"\")"="Data: Cleanup\nExit") -> ("States Out"=w273:string)  [unwired: 13 in]
            n134 = call <vilib>:"Add State(s) to Queue__JKI_lib_State_Machine.vi"("State(s) in Front (\"\")"=w273, "State(s) in (\"\")"=w278) -> ("States Out"=w277:string)  [unwired: 13 in]
          }
          frame "---------- API ----------" {
            # "#CSM \"Category Seperator\"\nDo not put any code in this frame."
          }
          frame "API: API1" {
            # "#CSM API Example\nCopy/Rename this case for your own API"
            # "#CSM Response\nConnect this to return the response of your API"
            # "#CSM >> Msg/Rep's CSM >>\nIf you need to tell who triggered this state , use this string. If it's this case itself, this string is \"\"."
            # "#CSM >> Arguments >>\nDeal with the parameter if any"
          }
          frame "API: API2" {
            # "#CSM API Example\nCopy/Rename this case for your own API"
            # "unpack Hex String  to Variant\nif complex parameter is needed."
            n135 = call "CSM - Convert HexStr to Data.vi"("HEX String"=w287) -> ()  [unwired: 7 in, 2 out]
            n136 = disable-structure shown="Disabled" {
              disable-tunnel: [w291 "API2 Response"] -> w286
              frame Disabled {
                # "pack variant to hexstr \nif complex response is needed."
                # "complex Response"
                n137 = call "CSM - Convert Data to HexStr.vi"() -> ("HEX String (0-9,A-F)"=w291:string)  [unwired: 9 in]
              }
              frame Enabled {
              }
            }
          }
          frame "---------- Action ----------" {
            # "#CSM \"Category Seperator\"\nDo not put any code in this frame."
            n138 = call <vilib>:"Add State(s) to Queue__JKI_lib_State_Machine.vi"("State(s) in (\"\")"=w296) -> ("States Out"=w295:string)  [unwired: 14 in]
          }
          frame "Action: action1" {
            # "#CSM \"Internal State\"\nThis category is used for holding internal states"
            n139 = call <vilib>:"Add State(s) to Queue__JKI_lib_State_Machine.vi"("State(s) in (\"\")"=w300) -> ("States Out"=w299:string)  [unwired: 14 in]
          }
          frame "Action: action2" {
            # "#CSM \"Internal State\"\nThis category is used for holding internal states"
            n140 = call <vilib>:"Add State(s) to Queue__JKI_lib_State_Machine.vi"("State(s) in (\"\")"=w304) -> ("States Out"=w303:string)  [unwired: 14 in]
          }
        }
      }
      n141 = flat-sequence {
        tunnel: w17 -> [w319]
        tunnel: [w316] -> w19
        tunnel: w16 -> [w313]
        tunnel: [w310] -> w18
        tunnel: w7 -> [w306]
        tunnel: w19 -> [w322]
        tunnel: [w322] -> w15
        tunnel: [w321] -> w14
        tunnel: w18 -> [w320]
        frame #0 {
          n142 = call "InitCSMs.vi"("Enable building lvlibp?"=FALSE, "testcase-CSMStatus in"=w319) -> ("error out"=w311:errorcluster, "testcase-CSMStatus out"=w317:refnum<class "testcase-CSMBroadcast.lvclass">)  [unwired: 8 in]
          n143 = Unbundle By Name(w311) -> ("status"=w315:bool)
          n144 = call "CSM - Wait and Send Message for Reply.vi"("State"="Macro: Exit", "Target Module"=w306) -> ("error out"=w307:errorcluster)  [unwired: 10 in, 3 out]
          n145 = call <vilib>:"Clear Errors.vi"("error in (no error)"=w307) -> ("error out"=w305:errorcluster)  [unwired: 5 in, 1 out]
          n146 = Not(x=w315) -> (.not. x?=w309:bool)
          n147 = call-dynamic "passIf.vi"("message (\"\")"="initCSMs.vi error" ("message (\"\")"), "pass"=w309, "TestCase in"=w317) -> ("error out"=w312:errorcluster, "TestCase out"=w316:refnum<class "testcase-CSMBroadcast.lvclass">)  [unwired: 7 in]
          n148 = Merge Errors(w313, w312, w311, w305) -> (w310:errorcluster)
        }
        frame #1 {
          n149 = call "CSM - Drop Broadcast Registry.vi"() -> ("error out"=w323:errorcluster)  [unwired: 15 in]
          n150 = Merge Errors(w320, w323) -> (w321:errorcluster)
        }
      }
    }
    frame Disabled {
      # "skip test result while test is under development"
      n151 = call <vilib>:"skip.vi"("error in (no error)"=w402, "TestCase in"=w405) -> ("error out"=w404:errorcluster, "TestCase out"=w403:refnum<class "testcase-CSMBroadcast.lvclass">)  [unwired: 8 in]
    }
  }
  "error out" <- w4
  "TestCase out" <- w2
